vi "DSF.Memory.Pointer.Array.Set Element Count.vi"(8 "error in (no error)":errorcluster, 10 "element count":u64 format="%d elements", 11 "Array Pointer in":refnum<class "DSF.Memory.Pointer.Array.lvclass">) -> (0 "error out":errorcluster, 3 "Array Pointer out":refnum<class "DSF.Memory.Pointer.Array.lvclass">)   [LabVIEW 2016, in "DSF.Memory.lvlib" / "DSF.Memory.Pointer.Array.lvclass"]
uses:
  DSF.Memory.Pointer.Array.lvclass
  DSF.Memory.Pointer.Array.lvclass/DSF.Memory.Pointer.Array.ctl
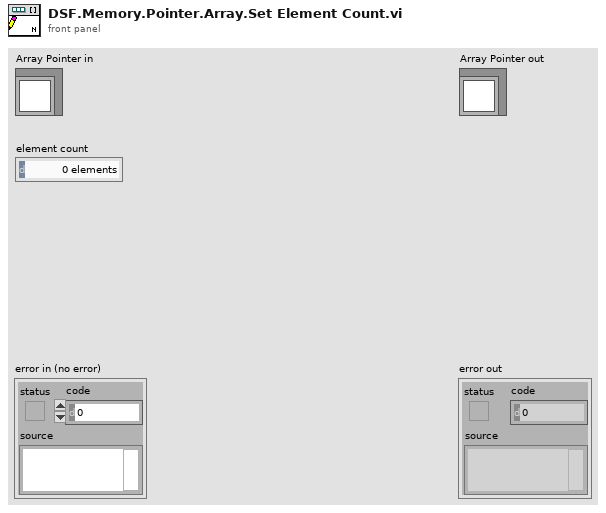
[diagram p1: front panel]
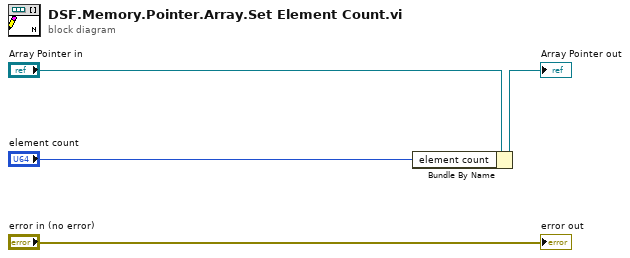
[diagram p0: block diagram]
diagram:
  n1 = Bundle By Name(cluster="Array Pointer in", "element count"="element count") -> (→"Array Pointer out":refnum<class "DSF.Memory.Pointer.Array.lvclass">)
  "error out" <- "error in (no error)"
